vi "Arm Scale.vi"(1 "Motor":enum16{"Base", "Shoulder", "Elbow", "Claw"}(ring), 2 "Angle in Particular Range (%)":u8(slide) scale=0.0..100.0) -> (0 "PWM":u16(slide) scale=500.0..2500.0)   [LabVIEW 2015]
panel:
  out "Deg":u16(slide) scale=0.0..180.0
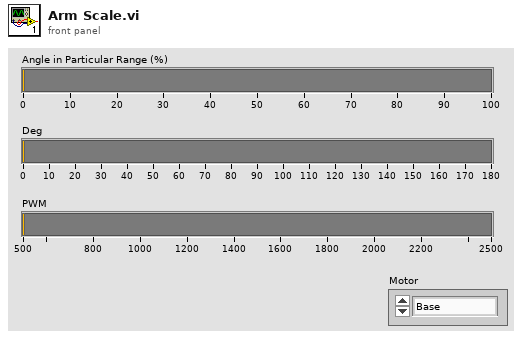
[diagram p1: front panel]
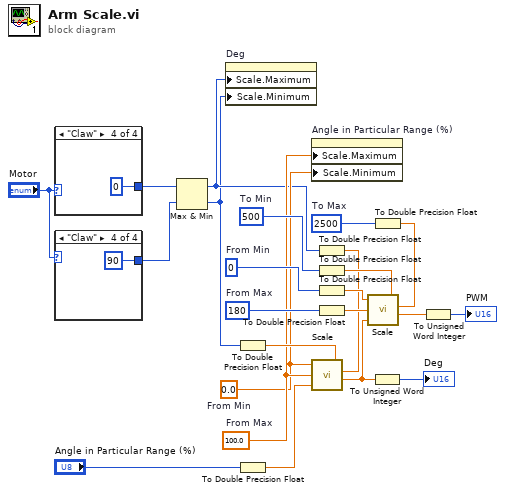
[diagram p0: block diagram]
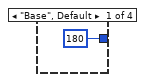
[diagram p2: hidden frame]
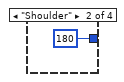
[diagram p3: hidden frame]
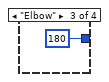
[diagram p4: hidden frame]
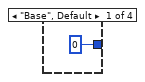
[diagram p5: hidden frame]
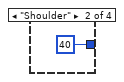
[diagram p6: hidden frame]
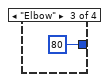
[diagram p7: hidden frame]
diagram:
  w18 = u64 2500  # To Max
  w17 = u64 500  # To Min
  w19 = u64 180  # From Max
  w16 = u64 0  # From Min
  w6 = 100.0  # From Max
  w5 = 0.0  # From Min
  n1 = case shown="\"Claw\"" "Motor" {
    tunnel: [0 40 80 0] -> w9
    frame "Base", Default {
    }
    frame "Shoulder" {
    }
    frame "Elbow" {
    }
    frame "Claw" {
    }
  }
  n2 = case shown="\"Claw\"" "Motor" {
    tunnel: [180 180 180 90] -> w8
    frame "Base", Default {
    }
    frame "Shoulder" {
    }
    frame "Elbow" {
    }
    frame "Claw" {
    }
  }
  n3 = Max & Min(x=w9, y=w8) -> (max(x,y)=w4:i32, min(x,y)=w3:i32)
  n4 = property on="Deg" class="Slide (strict)"("Scale.Maximum"=w4, "Scale.Minimum"=w3) -> ()  [unwired: 2 in, 2 out]
  n5 = To Double Precision Float(number=w3) -> (double precision float=w13:dbl)
  n6 = To Double Precision Float(number="Angle in Particular Range (%)") -> (double precision float=w12:dbl)
  n7 = property on="Angle in Particular Range (%)" class="Slide (strict)"("Scale.Maximum"=w6, "Scale.Minimum"=w5) -> ()  [unwired: 2 in, 2 out]
  n8 = To Double Precision Float(number=w4) -> (double precision float=w14:dbl)
  n9 = call "Scale.vi"("From Min"=w5, "From Max"=w6, "Input Val"=w12, "To Min"=w13, "To Max"=w14) -> ("Output val"=w1:dbl)  [unwired: 1 out]
  n10 = To Double Precision Float(number=w17) -> (double precision float=w22:dbl)
  n11 = To Double Precision Float(number=w16) -> (double precision float=w21:dbl)
  n12 = To Double Precision Float(number=w19) -> (double precision float=w20:dbl)
  n13 = To Unsigned Word Integer(number=w1) -> (unsigned 16bit integer=→"Deg":u16)
  n14 = To Double Precision Float(number=w18) -> (double precision float=w23:dbl)
  n15 = call "Scale.vi"("From Min"=w21, "From Max"=w20, "Input Val"=w1, "To Min"=w22, "To Max"=w23) -> ("Output val"=w15:dbl)  [unwired: 1 out]
  n16 = To Unsigned Word Integer(number=w15) -> (unsigned 16bit integer=→"PWM":u16)
